vi "CheckpointMeasurementDeviceReady.vi"(0 "Scanner IN":bool, 1 "Koheras laser IN":bool, 2 "CTIOTF IN":bool, 3 "Andor IN":bool, 5 "error in":errorcluster) -> (14 "PointMeasurementDeviceReady":bool, 19 "error out":errorcluster)   [LabVIEW 2011]
panel:
  in  "heidenhain":bool
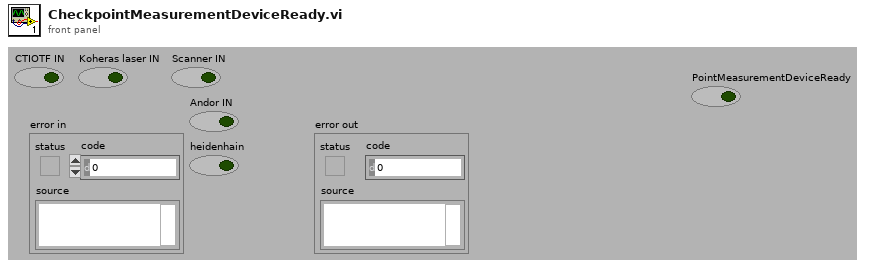
[diagram p1: front panel]
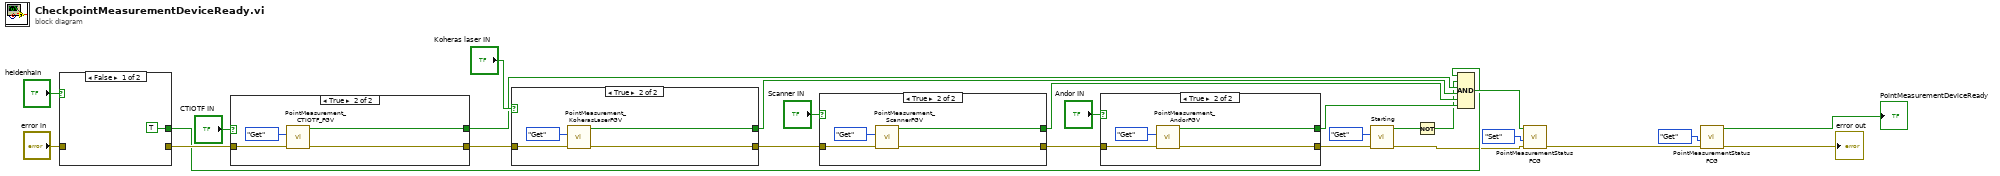
[diagram p0: block diagram]
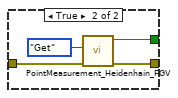
[diagram p2: hidden frame]
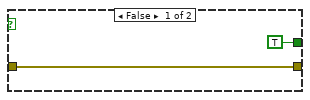
[diagram p3: hidden frame]
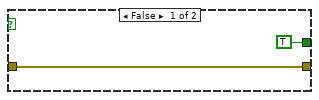
[diagram p4: hidden frame]
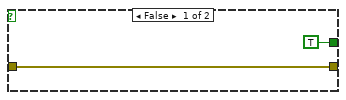
[diagram p5: hidden frame]
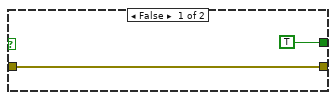
[diagram p6: hidden frame]
diagram:
  n1 = case shown="False" "heidenhain" {
    tunnel: "error in" -> [_ w30]
    tunnel: [_ w29] -> w4
    tunnel: [TRUE ("Get") w28] -> w2
    frame False {
    }
    frame True {
      n2 = call "PointMeasurement_Heidenhain_FGV.vi"("error in"=w30, "Set_Get"=enum16{"Set", "Get"}."Get") -> ("error out"=w29:errorcluster, "Get"=w28:bool)  [unwired: 8 in]
    }
  }
  n3 = case shown="True" "CTIOTF IN" {
    tunnel: w4 -> [w32 w36]
    tunnel: [w32 w35] -> w25
    tunnel: [TRUE ("Get") w34] -> w19
    frame False {
    }
    frame True {
      n4 = call "PointMeasurement_CTIOTF_FGV.vi"("error in"=w36, "Set_Get"=enum16{"Set", "Get"}."Get") -> ("error out"=w35:errorcluster, "Get"=w34:bool)  [unwired: 8 in]
    }
  }
  n5 = case shown="True" "Koheras laser IN" {
    tunnel: [w38 w42] -> w24
    tunnel: w25 -> [w38 w41]
    tunnel: [TRUE ("Get") w40] -> w20
    frame False {
    }
    frame True {
      n6 = call "PointMeasurement_KoherasLaserFGV.vi"("error in"=w41, "Set_Get"=enum16{"Set", "Get"}."Get") -> ("error out"=w42:errorcluster, "Get"=w40:bool)  [unwired: 8 in]
    }
  }
  n7 = case shown="True" "Scanner IN" {
    tunnel: w24 -> [w44 w48]
    tunnel: [w44 w47] -> w18
    tunnel: [TRUE ("Get") w46] -> w21
    frame False {
    }
    frame True {
      n8 = call "PointMeasurement_ScannerFGV.vi"("error in"=w48, "Set_Get"=enum16{"Set", "Get"}."Get") -> ("error out"=w47:errorcluster, "Get"=w46:bool)  [unwired: 8 in]
    }
  }
  n9 = case shown="True" "Andor IN" {
    tunnel: w18 -> [w50 w54]
    tunnel: [w50 w53] -> w9
    tunnel: [TRUE ("Get") w52] -> w17
    frame False {
    }
    frame True {
      n10 = call "PointMeasurement_AndorFGV.vi"("error in"=w54, "Set_Get"=enum16{"Set", "Get"}."Get") -> ("error out"=w53:errorcluster, "Get"=w52:bool)  [unwired: 8 in]
    }
  }
  n11 = call "Starting.vi"("error in"=w9, "Set_Get"=enum16{"Set", "Get"}."Get") -> ("error out"=w1:errorcluster, "Get"=w7:bool)  [unwired: 8 in]
  n12 = Not(x=w7) -> (.not. x?=w8:bool)
  n13 = Compound Arithmetic op=AND(w2, w8, w19, w20, w21, w17) -> (w6:bool)
  n14 = call "PointMeasurementStatusFCG.vi"("error in"=w1, "Set_Get"=enum16{"Set", "Get"}."Set", "Value"=w6) -> ("error out"=w14:errorcluster)  [unwired: 7 in, 1 out]
  n15 = call "PointMeasurementStatusFCG.vi"("error in"=w14, "Set_Get"=enum16{"Set", "Get"}."Get") -> ("error out"=→"error out":errorcluster, "Get"=→"PointMeasurementDeviceReady":bool)  [unwired: 8 in]
